vi "get condition.vi"(11 "Report Cluster":refnum<vi>) -> (3 "Condition":string)   [LabVIEW 2015]
uses:
  controls/Query for report Cluster.ctl
  controls/Type.ctl
  controls/Back to Business.ctl
  controls/Declined.ctl
  controls/Program.ctl
  controls/Case Status.ctl
  controls/Date to query in report.ctl
  controls/Amount in query for report.ctl
panel:
  in  "Report Cluster 2":T1 {"Business Replay date"."From :" format="%<%d/%m/%y>T"; "Business Replay date"."To :" format="%<%d/%m/%y>T"; "Next Review date"."From :" format="%<%d/%m/%y>T"; "Next Review date"."To :" format="%<%d/%m/%y>T"; "Stamped date"."From :" format="%<%d/%m/%y>T"; "Stamped date"."To :" format="%<%d/%m/%y>T"; "CAD submission date"."From :" format="%<%d/%m/%y>T"; "CAD submission date"."To :" format="%<%d/%m/%y>T"; "decline date"."From :" format="%<%d/%m/%y>T"; "decline date"."To :" format="%<%d/%m/%y>T"; "CAM date"."From :" format="%<%d/%m/%y>T"; "CAM date"."To :" format="%<%d/%m/%y>T"; "Pending risk visit date"."From :" format="%<%d/%m/%y>T"; "Pending risk visit date"."To :" format="%<%d/%m/%y>T"; "Back to business 3"."From :" format="%<%d/%m/%y>T"; "Back to business 3"."To :" format="%<%d/%m/%y>T"; "Back to business 2"."From :" format="%<%d/%m/%y>T"; "Back to business 2"."To :" format="%<%d/%m/%y>T"; "Back to business 1"."From :" format="%<%d/%m/%y>T"; "Back to business 1"."To :" format="%<%d/%m/%y>T"; "3rd login Date"."From :" format="%<%d/%m/%y>T"; "3rd login Date"."To :" format="%<%d/%m/%y>T"; "2nd login Date"."From :" format="%<%d/%m/%y>T"; "2nd login Date"."To :" format="%<%d/%m/%y>T"; "1st Login Date"."From :" format="%<%d/%m/%y>T"; "1st Login Date"."To :" format="%<%d/%m/%y>T"}
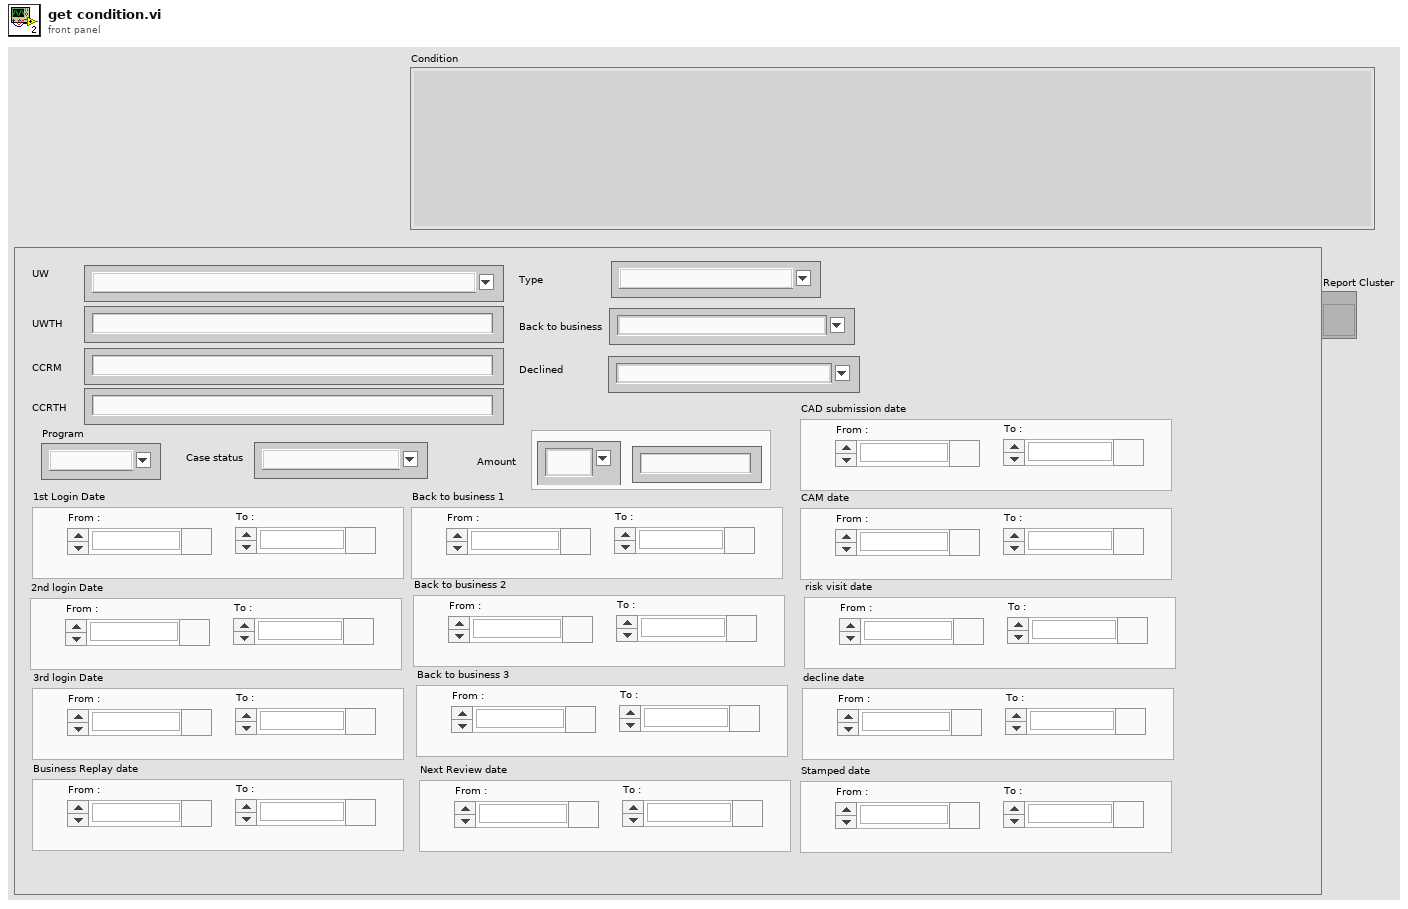
[diagram p1: front panel]
types:
  T1 = typedef "Query for report Cluster.ctl" = cluster{"UW":string, "UWTH":string, "CCRM":string, "CCRTH":string, "Type":T2, "Back to business":T3, "Declined":T4, "Program":T5, "Case status":T6, "1st Login Date":T7, "2nd login Date":T7, "3rd login Date":T7, "Business Replay date":T7, "Back to business 1":T7, "Back to business 2":T7, "Back to business 3":T7, "Next Review date":T7, "CAD submission date":T7, "CAM date":T7, "Pending risk visit date":T7, "decline date":T7, "Stamped date":T7, "Amount":T8, "Customer Number":string, "Customer Name":string, "Comment":string, "serial":string}
  T2 = typedef "Type.ctl" = string
  T3 = typedef "Back to Business.ctl" = string
  T4 = typedef "Declined.ctl" = string
  T5 = typedef "Program.ctl" = string
  T6 = typedef "Case Status.ctl" = string
  T7 = typedef "Date to query in report.ctl" = cluster{"To :":timestamp, "From : ":timestamp}
  T8 = typedef "Amount in query for report.ctl" = cluster{"Amount":string, "Comparison":string}
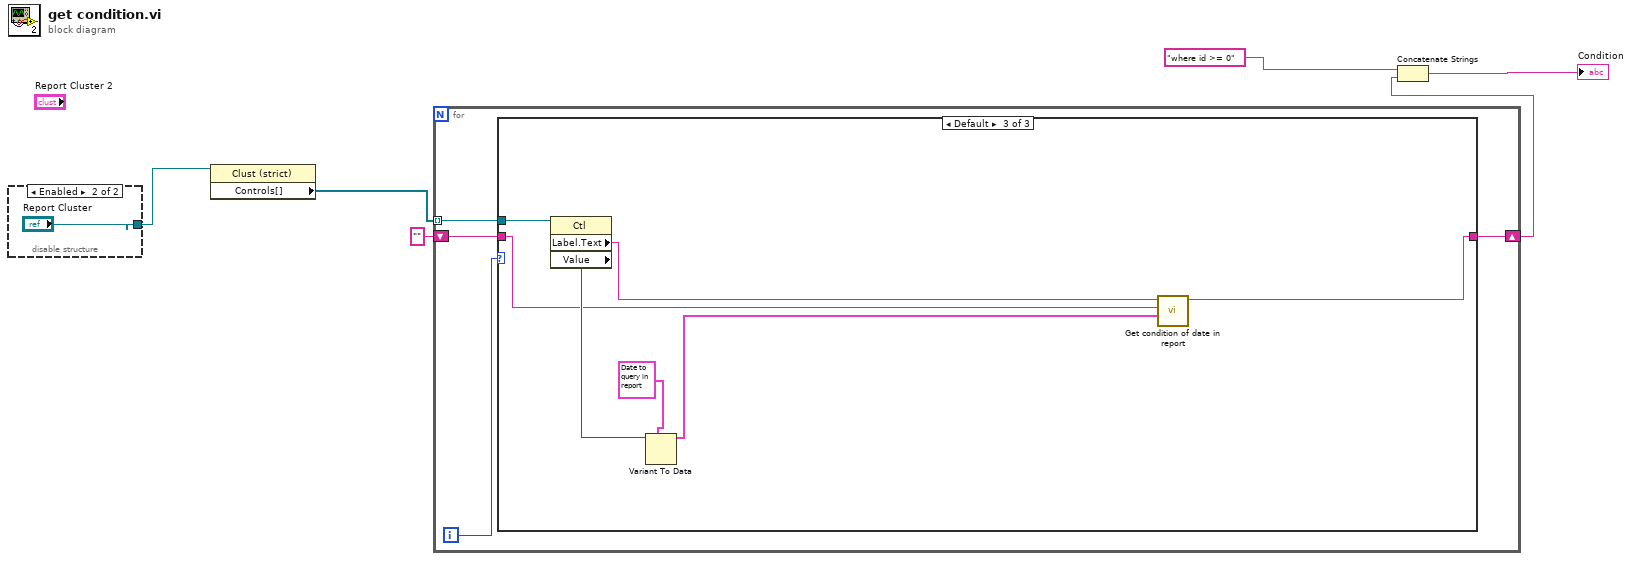
[diagram p0: block diagram]
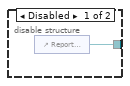
[diagram p2: hidden frame]
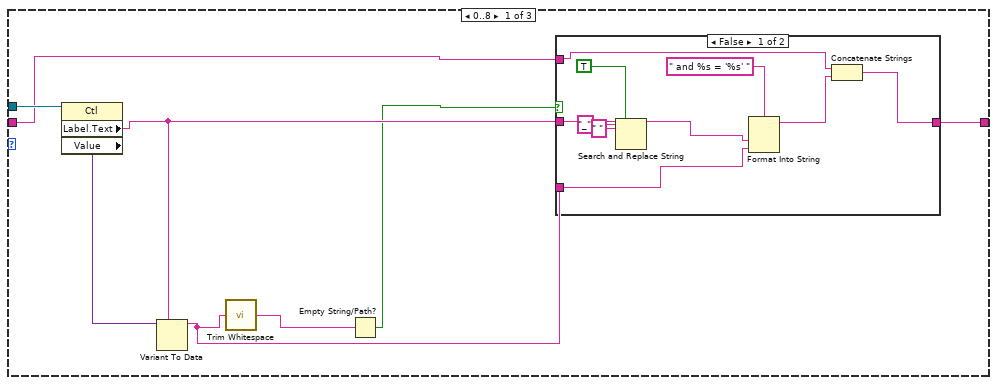
[diagram p3: hidden frame]
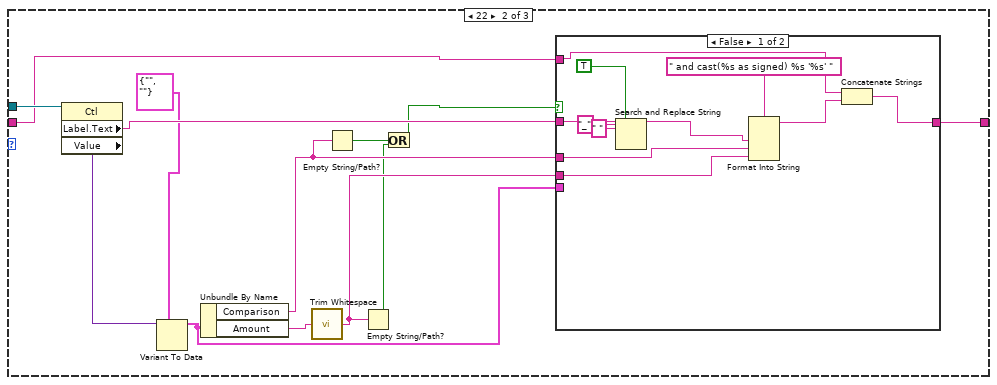
[diagram p5: hidden frame]
diagram:
  n1 = disable-structure shown="Enabled" {
    disable-tunnel: [w7 "Report Cluster"] -> w1
    frame Disabled {
      n2 = control-ref of="Report Cluster 2"() -> (w7:refnum<vi>)
    }
    frame Enabled {
    }
  }
  n3 = property class="Clust (strict)"(reference=w1) -> ("Controls[]"=w5:refnum<vi>[])  [unwired: 1 in, 2 out]
  n4 = for {
    tunnel: w5 -> [w11] mode=indexing
    shift-right: [w10] -> w3
    shift-left: "" -> [w9]
    i -> [w12]
    n5 = case shown="Default" w12 {
      tunnel: w11 -> [w20 w44 w63]
      tunnel: [w16 w41 w60] -> w10
      tunnel: w9 -> [w15 w40 w59]
      frame 0..8 {
        n6 = property class="Ctl"(reference=w20) -> ("Label.Text"=w18:string, "Value"=w19:variant)  [unwired: 1 in, 2 out]
        n7 = Variant To Data(type=w18, Variant=w19) -> (data=w14:string)  [unwired: 1 in, 1 out]
        n8 = call <vilib>:"Trim Whitespace.vi"("string"=w14) -> ("trimmed string"=w13:string)  [unwired: 1 in]
        n9 = Empty String/Path?(string/path=w13) -> (empty?=w17:bool)
        n10 = case shown="False" w17 {
          tunnel: w18 -> [w29 _]
          tunnel: [w22 w31] -> w16
          tunnel: w15 -> [w24 w31]
          tunnel: w14 -> [w21 _]
          frame False {
            n11 = Search and Replace String(replace all?=TRUE ("replace all? (F)"), input string=w29, search string=" ", replace string="_" ("replace string (\"\")")) -> (result string=w25:string)  [unwired: 4 in, 3 out]
            n12 = Format Into String(format string=" and %s = '%s' ", w25, w21) -> (resulting string=w23:string)  [unwired: 2 in, 1 out]
            n13 = Concatenate Strings(w24, w23) -> (w22:string)
          }
          frame True {
          }
        }
      }
      frame 22 {
        n14 = property class="Ctl"(reference=w44) -> ("Label.Text"=w42:string, "Value"=w43:variant)  [unwired: 1 in, 2 out]
        n15 = Variant To Data(type=T8 {"Amount"="", "Comparison"=""} ("Amount Condition"), Variant=w43) -> (data=w38:T8)  [unwired: 1 in, 1 out]
        n16 = Unbundle By Name(w38) -> ("Comparison"=w35:string, "Amount"=w37:string)
        n17 = call <vilib>:"Trim Whitespace.vi"("string"=w37) -> ("trimmed string"=w36:string)  [unwired: 1 in]
        n18 = Empty String/Path?(string/path=w35) -> (empty?=w34:bool)
        n19 = Empty String/Path?(string/path=w36) -> (empty?=w33:bool)
        n20 = Or(x=w34, y=w33) -> (x .or. y?=w32:bool)
        n21 = case shown="False" w32 {
          tunnel: w42 -> [w54 _]
          tunnel: [w47 w56] -> w41
          tunnel: w40 -> [w49 w56]
          tunnel: w38 -> [_ _]
          tunnel: w35 -> [w46 _]
          tunnel: w36 -> [w45 _]
          frame False {
            n22 = Search and Replace String(replace all?=TRUE ("replace all? (F)"), input string=w54, search string=" ", replace string="_" ("replace string (\"\")")) -> (result string=w50:string)  [unwired: 4 in, 3 out]
            n23 = Format Into String(format string=" and cast(%s as signed) %s '%s' ", w50, w46, w45) -> (resulting string=w48:string)  [unwired: 2 in, 1 out]
            n24 = Concatenate Strings(w49, w48) -> (w47:string)
          }
          frame True {
          }
        }
      }
      frame Default {
        n25 = property class="Ctl"(reference=w63) -> ("Label.Text"=w61:string, "Value"=w62:variant)  [unwired: 1 in, 2 out]
        n26 = Variant To Data(type=T7 {"To :"=timestamp(0 s since 1904-01-01), "From : "=timestamp(0 s since 1904-01-01)} ("Date"), Variant=w62) -> (data=w58:T7)  [unwired: 1 in, 1 out]
        n27 = call "Get condition of date in report.vi"("Date"=w58, "Intial condition"=w59, "Date Label"=w61) -> ("Condition"=w60:string)  [unwired: 8 in]
      }
    }
  }
  n28 = Concatenate Strings("where id >= 0", w3) -> (→"Condition":string)
